vi "Read Voltage Hum.vi"(6 "Error In":errorcluster) -> (0 "Error Out":errorcluster, 3 "Porcentaje":dbl)   [LabVIEW 2016]
doc: "This VI is used in the LabVIEW Core 1 & 2 courses.\n\nThis VI simulates taking voltage readings from a DAQ board. Use this VI to replace the DAQ Assistant Express VI in any temperature reading exercises in this course. This VI is used as a subVI in all (Demo) exercises."
uses:
  <vilib>/gmath/statdist.llb/Normal Random.vi
  <vilib>/gmath/NI_Gmath.lvlib
panel:
  out "normal random data":dbl[](array[numeric])
  # "This VI is a demo version of a VI that reads the voltage on Device 1, channel 0.  When scaled by 100, value can represent temperature."
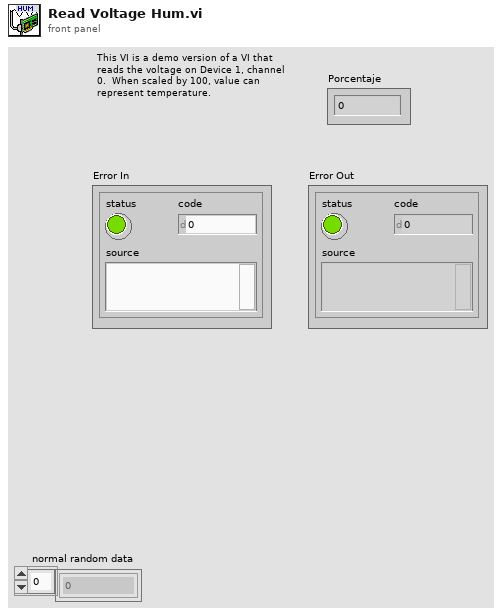
[diagram p1: front panel]
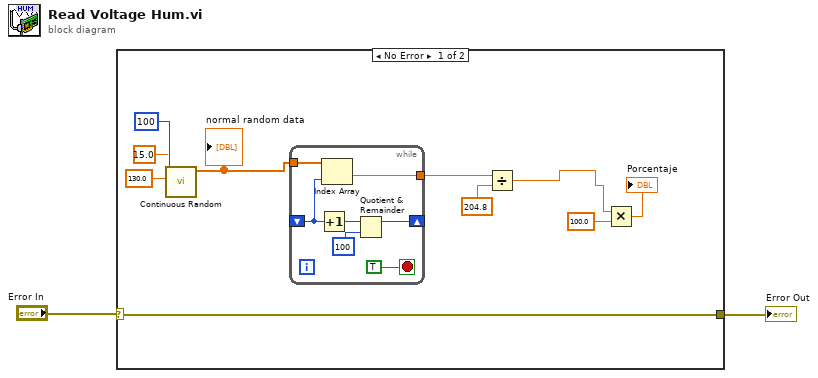
[diagram p0: block diagram]
diagram:
  n1 = case shown="No Error" "Error In" {
    selector: "Error In" -> [w10 w20]
    tunnel: [w10 w20] -> w2
    frame No Error {
      n2 = call-poly <vilib>:"Continuous Random.vi"("std"=15.0, "mean"=130.0, "samples"=100) -> ("normal random data"=w9:dbl[])  [unwired: 7 in, 1 out]
      "normal random data" <- w9
      n3 = while {
        tunnel: w9 -> [w14]
        tunnel: [w15] -> w11
        shift-left: _ -> [w19]
        shift-right: [w16] -> _
        stop <- TRUE stop-if-true
        n4 = Increment(x=w19) -> (x+1=w18:i32)
        n5 = Index Array(array=w14, index=w19) -> (element=w15:dbl)
        n6 = Quotient & Remainder(x=w18, y=100) -> (x-y*floor(x/y)=w16:i32)  [unwired: 1 out]
      }
      n7 = Divide(x=w11, y=204.8) -> (x/y=w3:dbl)
      n8 = Multiply(x=w3, y=100.0) -> (x*y=→"Porcentaje":dbl)
    }
    frame Error {
    }
  }
  "Error Out" <- w2
